vi "MU Calibration Set Current Nonius Track Offset Table.vi"(8 "error in (no error)":errorcluster, 10 "optimizedNoniusTrackOffsetTable":cluster{"spoBase":i8, "spoN":i8[]}={"spoBase"=0, "spoN"=[0, 0, 0, 0, 0, 0, 0, 0, 0, 0, 0, 0, 0, 0, 0, 0]}, 11 "CalibrationHandle":T1) -> (0 "error out (no error)":errorcluster, 3 "function return":bool)   [LabVIEW 2017, in "MU_3SL_interface.lvlib"]
uses:
  MU_3SL_interface.lvlib
  handles/CalibrationHandle.ctl
  lib/MU_3SL_interface.dll
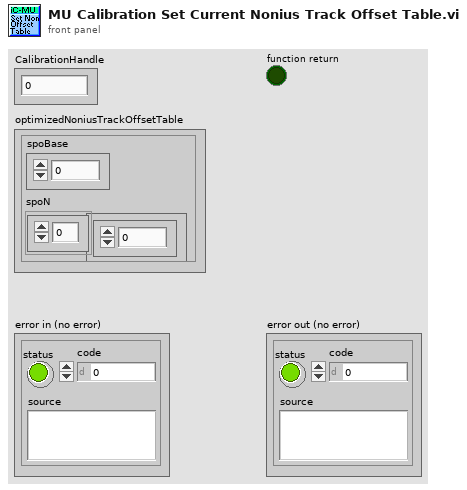
[diagram p1: front panel]
types:
  T1 = typedef "MU_3SL_interface.lvlib/CalibrationHandle.ctl" = u64
  T2 = cluster{"[0]":i8, "[1]":i8, "[2]":i8, "[3]":i8, "[4]":i8, "[5]":i8, "[6]":i8, "[7]":i8, "[8]":i8, "[9]":i8, "[10]":i8, "[11]":i8, "[12]":i8, "[13]":i8, "[14]":i8, "[15]":i8, "[16]":i8}
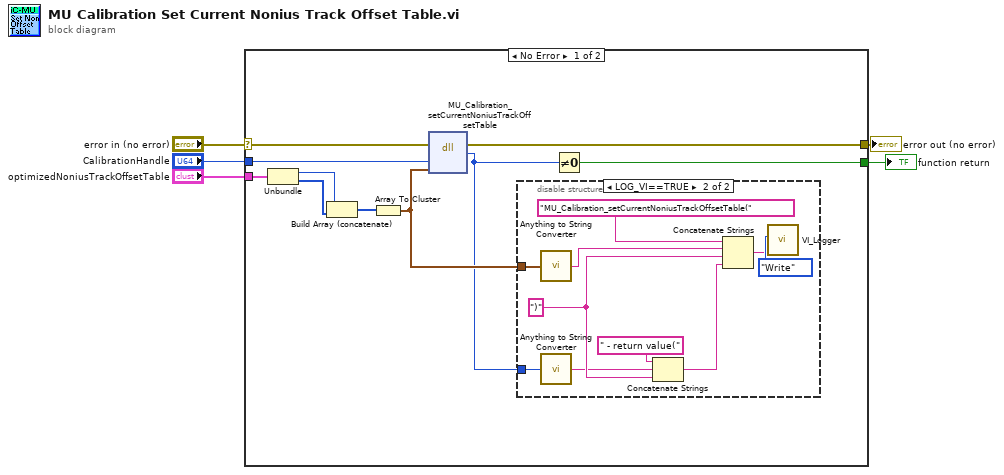
[diagram p0: block diagram]
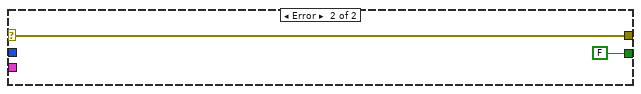
[diagram p3: hidden frame]
diagram:
  n1 = case shown="No Error" "error in (no error)" {
    selector: "error in (no error)" -> [w15 w27]
    tunnel: [w13 w27] -> w5
    tunnel: "CalibrationHandle" -> [w14 _]
    tunnel: "optimizedNoniusTrackOffsetTable" -> [w12 _]
    tunnel: [w6 FALSE] -> w1
    frame No Error {
      n2 = Unbundle(w12) -> ("spoBase"=w11:i8, "spoN"=w10:i8[])
      n3 = Build Array (concatenate)(w11, w10) -> (w9:i8[])
      n4 = Array To Cluster(array=w9) -> (cluster=w8:T2)
      n5 = dll-call lib="C:/Users/bes/AppData/Roaming/work/mu_9so/icsubmodules/soft_mu_3sl_master/lv_interface/lib/MU_3SL_interface**.*" fn="MU_Calibration_setCurrentNoniusTrackOffsetTable"(error in=w15, "calibrationHandle"=w14, "optimizedNoniusTrackOffsetTable"=w8) -> (error out=w13:errorcluster, "Return Value"=w7:u8)  [unwired: 4 in, 1 out]
      n6 = disable-structure shown="LOG_VI==TRUE" {
        disable-tunnel: w8 -> [_ w21]
        disable-tunnel: w7 -> [_ w18]
        frame condition #0 {
        }
        frame condition #1 (active) {
          w19 = ")" ("string")
          n7 = call "Anything to String Converter.vi"("anything"=w21) -> ("String"=w20:string)
          n8 = call "Anything to String Converter.vi"("anything"=w18) -> ("String"=w17:string)
          n9 = Concatenate Strings(" - return value(" ("string"), w17, w19) -> (w16:string)
          n10 = Concatenate Strings("MU_Calibration_setCurrentNoniusTrackOffsetTable(" ("Info in"), w20, w19, w16) -> (w23:string)
          n11 = call "VI_Logger.vi"("Action (Read)"=enum16{"Write", "Read"}."Write", "Info in"=w23) -> ()  [unwired: 8 in, 2 out]
        }
      }
      n12 = Not Equal To 0?(x=w7) -> (x != 0?=w6:bool)
    }
    frame Error {
    }
  }
  "error out (no error)" <- w5
  "function return" <- w1
